vi "CRYGet Print Unit.vi"(6 "dB ref":dbl, 8 "Unit":string, 9 "Common dB #":u16, 10 "Common dB":string, 11 "Scale":u16(slide)) -> (3 "Print Unit":string)   [LabVIEW 2013]
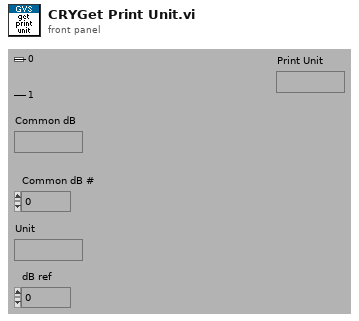
[diagram p1: front panel]
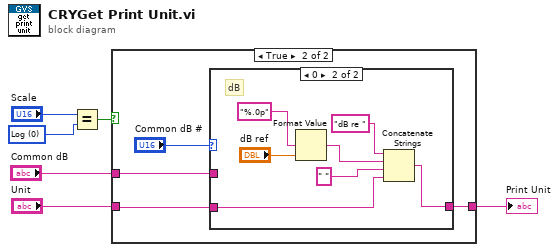
[diagram p0: block diagram]
diagram:
  w4 = u16 0 items=["Log", "Linear"] ("Scale")
  n1 = Equal?(x="Scale", y=w4) -> (x = y?=w6:bool)
  n2 = case shown="True" w6 {
    tunnel: "Unit" -> [w7 w11]
    tunnel: [w7 w10] -> w1
    tunnel: "Common dB" -> [_ w8]
    frame False {
    }
    frame True {
      n3 = case shown="0" "Common dB #" {
        tunnel: w11 -> [_ w14]
        tunnel: [w12 w17] -> w10
        tunnel: w8 -> [w12 _]
        frame Default {
          # "Others"
        }
        frame 0 {
          # "dB"
          n4 = Format Value(format string="%.0p", value (0)="dB ref") -> (output string=w19:string)  [unwired: 1 in]
          n5 = Concatenate Strings("dB re " ("string"), w19, " " ("string"), w14) -> (w17:string)
        }
      }
    }
  }
  "Print Unit" <- w1
